vi "NI9234_driver.vi"(6 "Method NI9205":T2, 8 "error in":errorcluster, 10 "SET_NI9234":T1={"IEPE Current value (A)"=0.004, "Sensitivity ACC (mV/g)"=10200.0, "Sample Rate (Sample/sec)"=1000.0, "Samples per Loop"=1000, "file path (use dialog)"=path "", "File Name"="", "Save?"=FALSE} {"Samples per Loop" min=10 max=507900 step=1; "Sample Rate (Sample/sec)" min=400.0 max=51000.0 step=1.0; "Sensitivity ACC (mV/g)" min=5.0 max=500.0; "IEPE Current value (A)" format="%#_13g"}, 11 "Physical Channel":tag="Dev1/ai0") -> (0 "error out":errorcluster, 1 "task out":refnum<k21>, 2 "Actual Sample Rate":dbl=1000.0000111176631 format="%0.2f", 3 "data":waveform(dbl)[](array[waveform]))   [LabVIEW 2020]
uses:
  TYPEDEF/NI9234_TD_MethodNI9234.ctl
  TYPEDEF/SET_NI9234.ctl
  <vilib>/DAQmx/read.llb/DAQmx Read (Analog 1D Wfm NChan NSamp).vi
  <vilib>/DAQmx/configure/task.llb/DAQmx Configure Logging (TDMS).vi
  <vilib>/DAQmx/miscellaneous.llb/DAQmx Fill In Error Info.vi
panel:
  out "Max Acc Read":dbl
  out "min Acc Read":dbl
  out "Waveform Graph":waveform(dbl)[](graph)
  # "Acquired Data"
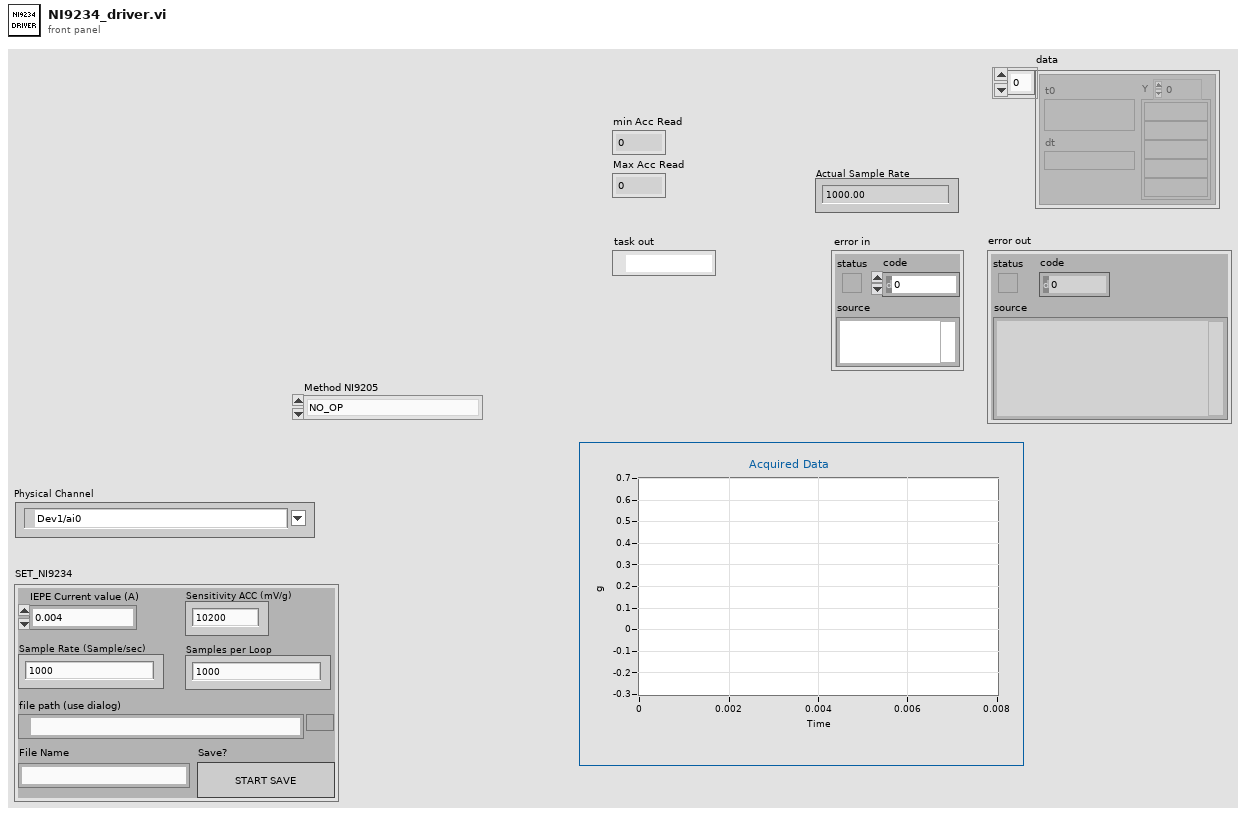
[diagram p1: front panel]
types:
  T1 = typedef "SET_NI9234.ctl" = cluster{"IEPE Current value (A)":dbl, "Sensitivity ACC (mV/g)":dbl, "Sample Rate (Sample/sec)":dbl, "Samples per Loop":i32, "file path (use dialog)":path, "File Name":string, "Save?":bool}
  T2 = typedef "NI9234_TD_MethodNI9234.ctl" = enum16{"NO_OP", "INIT", "SET", "GET", "CLOSE"}
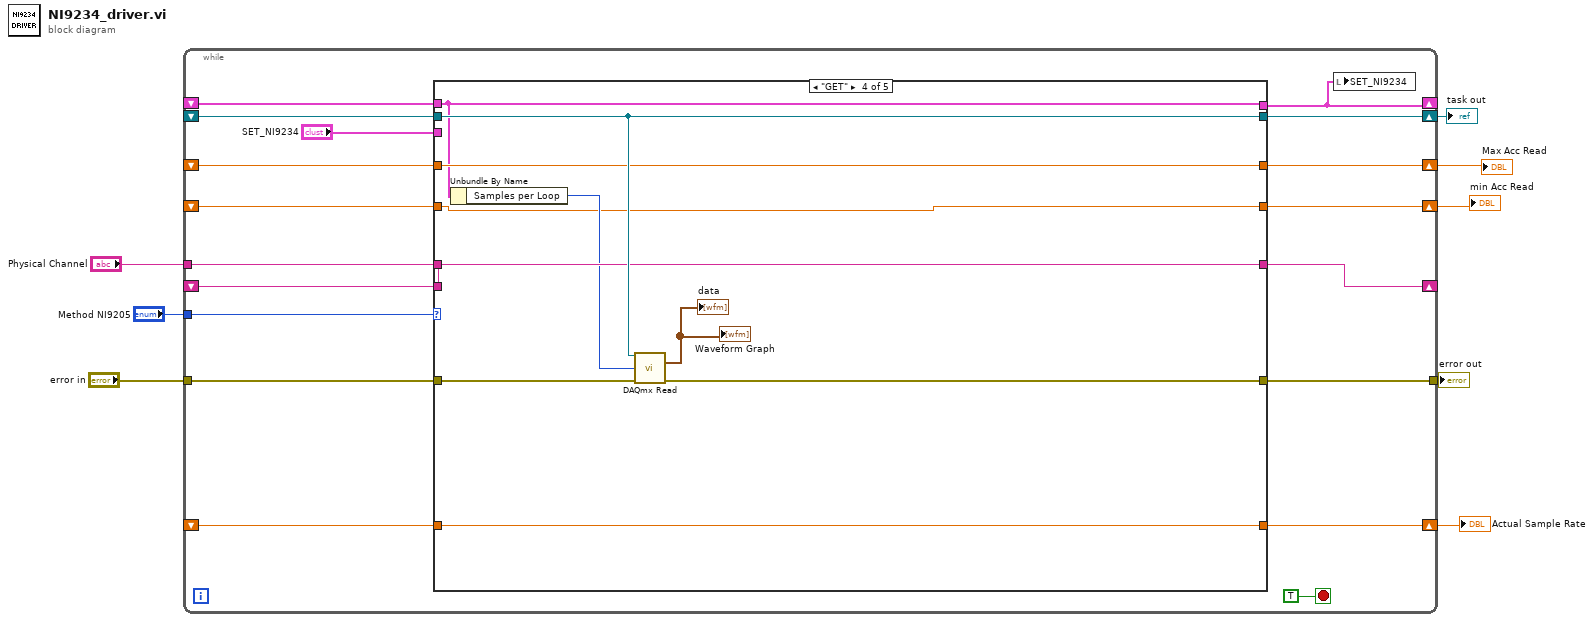
[diagram p0: block diagram]
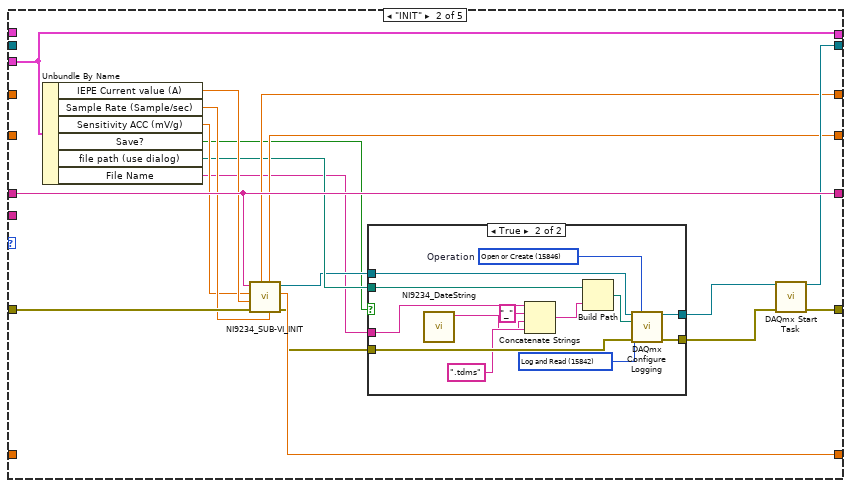
[diagram p3: hidden frame]
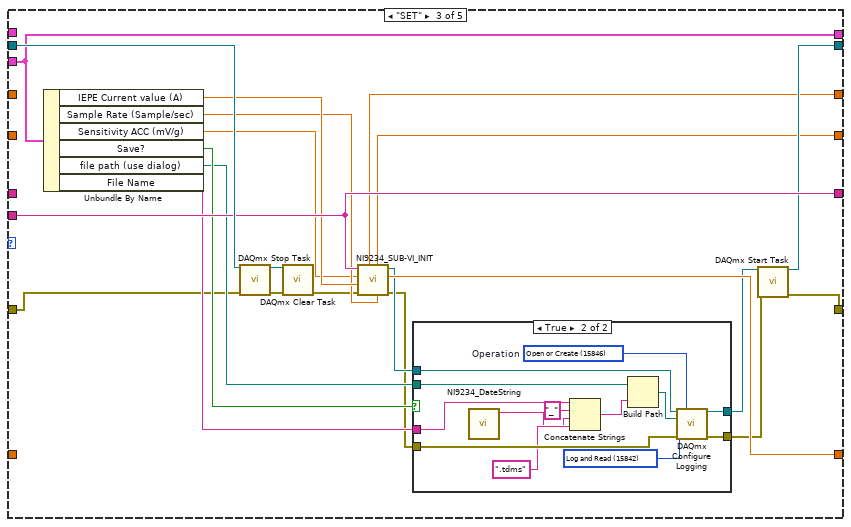
[diagram p5: hidden frame]
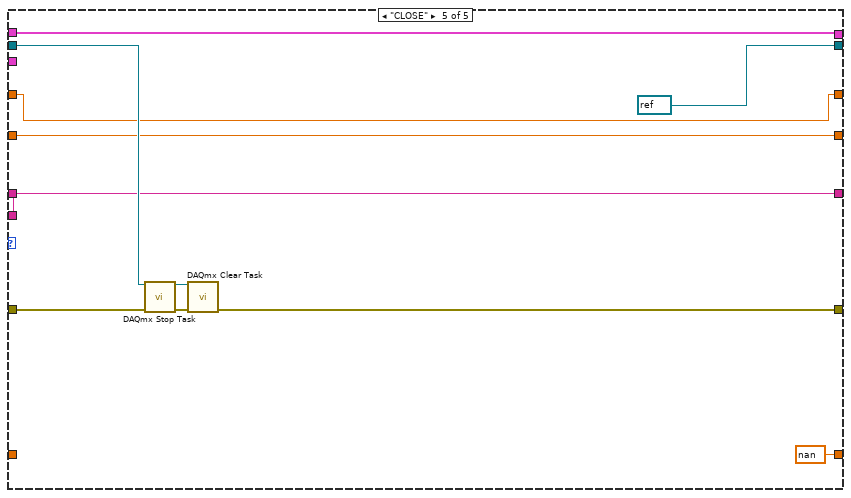
[diagram p7: hidden frame]
diagram:
  n1 = while {
    tunnel: "Method NI9205" -> [w25]
    tunnel: "error in" -> [w24]
    tunnel: [w23] -> w6
    tunnel: "Physical Channel" -> [w22]
    shift-right: [w21] -> w3
    shift-left: _ -> [w20]
    shift-right: [w19] -> w4
    shift-left: _ -> [w18]
    shift-right: [w17] -> _
    shift-left: _ -> [w16]
    shift-right: [w9] -> _
    shift-left: _ -> [w15]
    shift-right: [w13] -> w2
    shift-left: _ -> [w11]
    shift-right: [w12] -> w1
    shift-left: _ -> [w10]
    stop <- TRUE stop-if-true
    n2 = case shown="\"GET\"" w25 {
      tunnel: w24 -> [w32 w51 w68 w112 w123]
      tunnel: [w32 w45 w79 w111 w120] -> w23
      tunnel: w22 -> [_ w49 _ _ _]
      tunnel: [w33 w46 w80 w110 refnum<k21> refnum ("task out")] -> w21
      tunnel: w20 -> [w33 _ w86 w110 w122]
      tunnel: [w31 w50 w85 w109 nan ("Actual Sample Rate")] -> w19
      tunnel: w18 -> [w31 _ _ w109 _]
      tunnel: [w30 w49 w84 w108 w117] -> w17
      tunnel: w16 -> [w30 _ w84 w108 w117]
      tunnel: [w29 w42 w76 w104 w116] -> w9
      tunnel: w15 -> [w29 _ _ w104 w116]
      tunnel: "SET_NI9234" -> [_ w42 w76 _ _]
      tunnel: [w28 w44 w77 w106 w115] -> w13
      tunnel: [w27 w43 w78 w105 w114] -> w12
      tunnel: w11 -> [w28 _ _ w106 w115]
      tunnel: w10 -> [w27 _ _ w105 w114]
      frame "NO_OP", Default {
      }
      frame "INIT" {
        n3 = Unbundle By Name(w42) -> ("IEPE Current value (A)"=w48:dbl, "Sample Rate (Sample/sec)"=w47:dbl, "Sensitivity ACC (mV/g)"=w41:dbl, "Save?"=w37:bool, "file path (use dialog)"=w39:path, "File Name"=w36:string)
        n4 = call "NI9234_SUB-VI_INIT.vi"("Sample Rate"=w47, "error in"=w51, "IEPE Current value (A)"=w48, "Sensitivity (mV/g)"=w41, "Physical Channel"=w49) -> ("error out"=w40:errorcluster, "Actual Sample Rate"=w50:dbl, "task out"=w38:refnum<k21>, "min Acc Read"=w43:dbl, "Max Acc Read"=w44:dbl)  [unwired: 2 in]
        n5 = case shown="True" w37 {
          tunnel: w39 -> [_ w63]
          tunnel: w36 -> [_ w65]
          tunnel: w40 -> [w53 w60]
          tunnel: w38 -> [w52 w59]
          tunnel: [w52 w58] -> w35
          tunnel: [w53 w57] -> w34
          frame False {
          }
          frame True {
            w61 = 15842 items=["Off"=10231, "Log"=15844, "Log and Read"=15842] ("logging mode")
            w66 = 15846 items=["Open"=10437, "Open or Create"=15846, "Create or Replace"=15847, "Create"=15848]  # Operation
            n6 = call "NI9234_DateString.vi"() -> ("concatenated string"=w54:string)  [unwired: 11 in]
            n7 = Concatenate Strings(w65, "_" ("string"), w54, ".tdms" ("string")) -> (w64:string)
            n8 = Build Path(base path=w63, name or relative path=w64) -> (appended path=w62:path)
            n9 = call-poly <vilib>:"DAQmx Configure Logging.vi"("task/channels in"=w59, "operation"=w66, "file path"=w62, "logging mode"=w61, "error in"=w60) -> ("task out"=w58:refnum<k21>, "error out"=w57:errorcluster)  [unwired: 9 in]
          }
        }
        n10 = call <vilib>:"DAQmx Start Task.vi"("task/channels in"=w35, "error in"=w34) -> ("task out"=w46:refnum<k21>, "error out"=w45:errorcluster)  [unwired: 12 in]
      }
      frame "SET" {
        n11 = Unbundle By Name(w76) -> ("IEPE Current value (A)"=w83:dbl, "Sample Rate (Sample/sec)"=w82:dbl, "Sensitivity ACC (mV/g)"=w81:dbl, "Save?"=w75:bool, "file path (use dialog)"=w74:path, "File Name"=w73:string)
        n12 = call <vilib>:"DAQmx Stop Task.vi"("task/channels in"=w86, "error in"=w68) -> ("task out"=w87:refnum<k21>, "error out"=w88:errorcluster)  [unwired: 12 in]
        n13 = call <vilib>:"DAQmx Clear Task.vi"("task in"=w87, "error in"=w88) -> ("error out"=w72:errorcluster)  [unwired: 13 in]
        n14 = call "NI9234_SUB-VI_INIT.vi"("Sample Rate"=w82, "error in"=w72, "IEPE Current value (A)"=w83, "Sensitivity (mV/g)"=w81, "Physical Channel"=w84) -> ("error out"=w67:errorcluster, "Actual Sample Rate"=w85:dbl, "task out"=w71:refnum<k21>, "min Acc Read"=w78:dbl, "Max Acc Read"=w77:dbl)  [unwired: 2 in]
        n15 = case shown="True" w75 {
          tunnel: w74 -> [_ w100]
          tunnel: w73 -> [_ w102]
          tunnel: w67 -> [w90 w97]
          tunnel: w71 -> [w89 w96]
          tunnel: [w89 w95] -> w70
          tunnel: [w90 w94] -> w69
          frame False {
          }
          frame True {
            w98 = 15842 items=["Off"=10231, "Log"=15844, "Log and Read"=15842] ("logging mode")
            w103 = 15846 items=["Open"=10437, "Open or Create"=15846, "Create or Replace"=15847, "Create"=15848]  # Operation
            n16 = call "NI9234_DateString.vi"() -> ("concatenated string"=w91:string)  [unwired: 11 in]
            n17 = Concatenate Strings(w102, "_" ("string"), w91, ".tdms" ("string")) -> (w101:string)
            n18 = Build Path(base path=w100, name or relative path=w101) -> (appended path=w99:path)
            n19 = call-poly <vilib>:"DAQmx Configure Logging.vi"("task/channels in"=w96, "operation"=w103, "file path"=w99, "logging mode"=w98, "error in"=w97) -> ("task out"=w95:refnum<k21>, "error out"=w94:errorcluster)  [unwired: 9 in]
          }
        }
        n20 = call <vilib>:"DAQmx Start Task.vi"("task/channels in"=w70, "error in"=w69) -> ("task out"=w80:refnum<k21>, "error out"=w79:errorcluster)  [unwired: 12 in]
      }
      frame "GET" {
        n21 = Unbundle By Name(w104) -> ("Samples per Loop"=w107:i32)
        n22 = call-poly <vilib>:"DAQmx Read.vi"("task/channels in"=w110, "number of samples per channel"=w107, "error in"=w112) -> ("data"=→"Waveform Graph" →"data":waveform(dbl)[], "error out"=w111:errorcluster)  [unwired: 10 in, 1 out]
      }
      frame "CLOSE" {
        n23 = call <vilib>:"DAQmx Stop Task.vi"("task/channels in"=w122, "error in"=w123) -> ("task out"=w121:refnum<k21>, "error out"=w124:errorcluster)  [unwired: 12 in]
        n24 = call <vilib>:"DAQmx Clear Task.vi"("task in"=w121, "error in"=w124) -> ("error out"=w120:errorcluster)  [unwired: 13 in]
      }
    }
    n25 = local write "SET_NI9234"(w9) -> ()
  }
  "error out" <- w6
  "Actual Sample Rate" <- w4
  "task out" <- w3
  "Max Acc Read" <- w2
  "min Acc Read" <- w1
